vi "Set Cell Position.vi"(10 "Cell Position":T1, 11 "listbox in":refnum<class "listbox.lvclass">) -> (3 "listbox out":refnum<class "listbox.lvclass">)   [LabVIEW 2016, in "listbox.lvclass"]
uses:
  listbox.lvclass
  <vilib>/Utility/miscctls.llb/LVRowAndColumnTypeDef.ctl
  listbox.lvclass/listbox.ctl
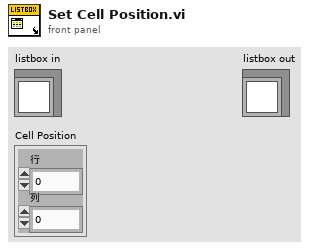
[diagram p1: front panel]
types:
  T1 = typedef "LVRowAndColumnTypeDef.ctl" = cluster{"Row":i32, "Column":i32}
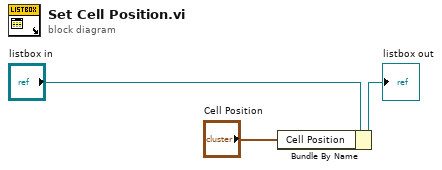
[diagram p0: block diagram]
diagram:
  n1 = Bundle By Name(cluster="listbox in", "Cell Position"="Cell Position") -> (→"listbox out":refnum<class "listbox.lvclass">)
